vi "TRHmeasurement.vi"() -> ()   [LabVIEW 2018]
panel:
  in  "Instrument":enum16{"AG34401A", "Arduino", "Manually"}(ring)
  in  "rel. Humidity [%] in":dbl
  in  "Temperature [°C] in":dbl
  in  "Write into text file":bool
  in  "stop":bool
  in  "Measurement delay [s]":u32=5
  out "Rel. Humidity [%]":dbl
  out "Temperature [°C]":dbl
  out "Max temperature [°C]":dbl
  out "Min temperature [°C]":dbl
  out "Max RH [%]":dbl
  out "Min RH [%]":dbl
  out "Last 10 measurements":string[][](table)
  out "Temp. & RH":cluster{dbl[], dbl[]}[](graph)
  out "Average temperature [°C]":dbl
  out "Average RH [%]":dbl
  out "Iteration start time":timestamp
  out "time":string
  out "error out":errorcluster
  in  "T&RH":refnum<visa-resource-name>="COM4"
  in  "error in":errorcluster
  in  "Select folder to save data":path=path "C:/Users/itkstriplabview5/Documents"
  out "output file refnum":refnum<file>
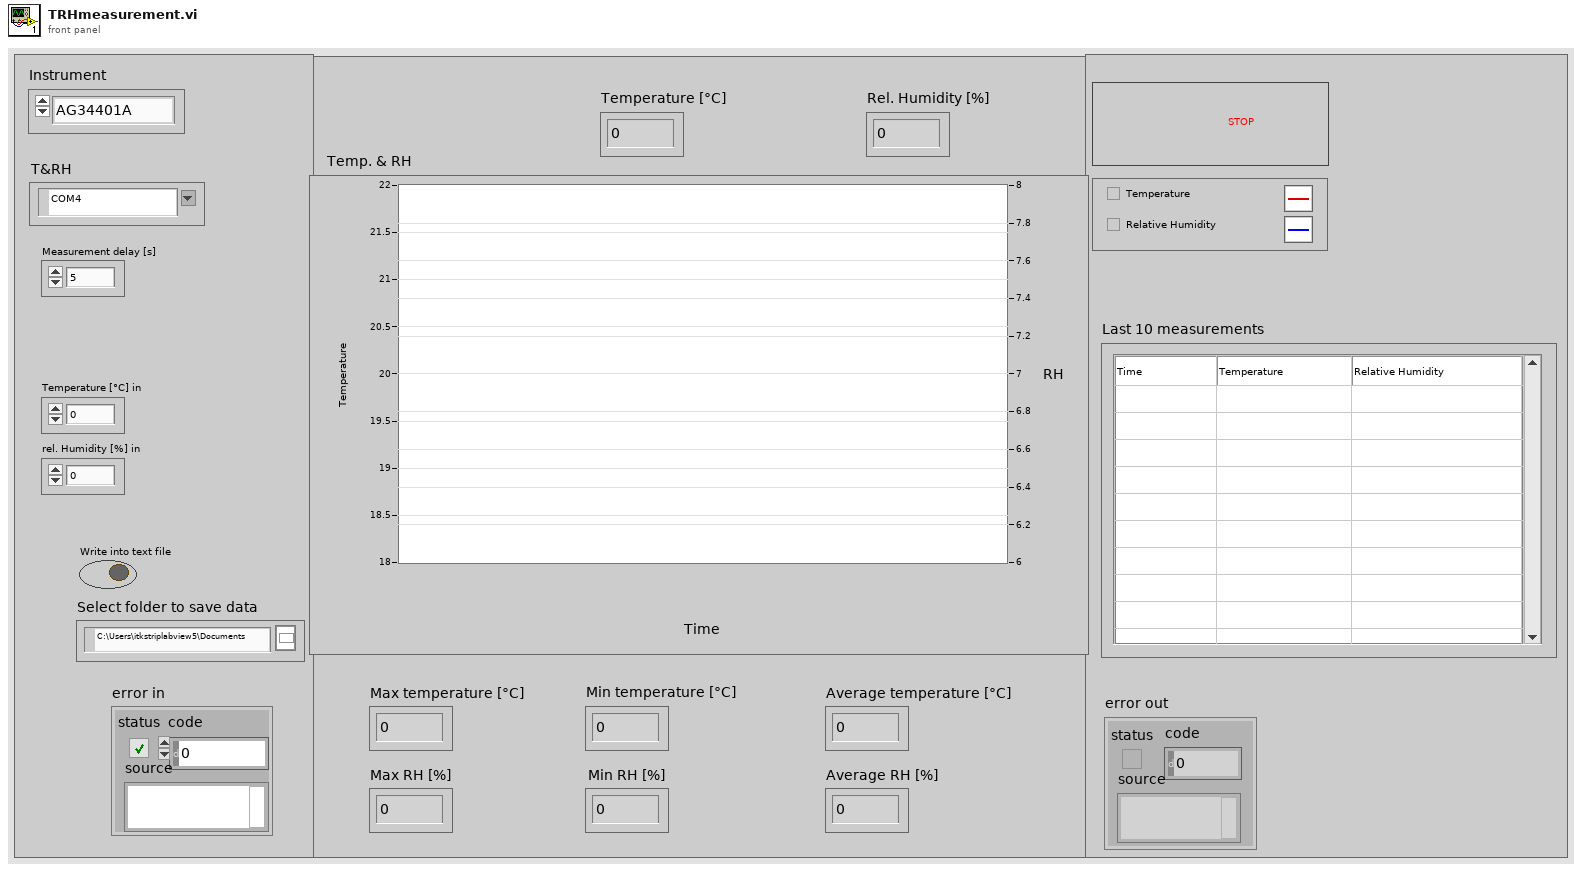
[diagram p1: front panel]
types:
  T1 = enum16{"open", "replace", "create", "open or create", "replace or create", "replace or create with confirmation"}
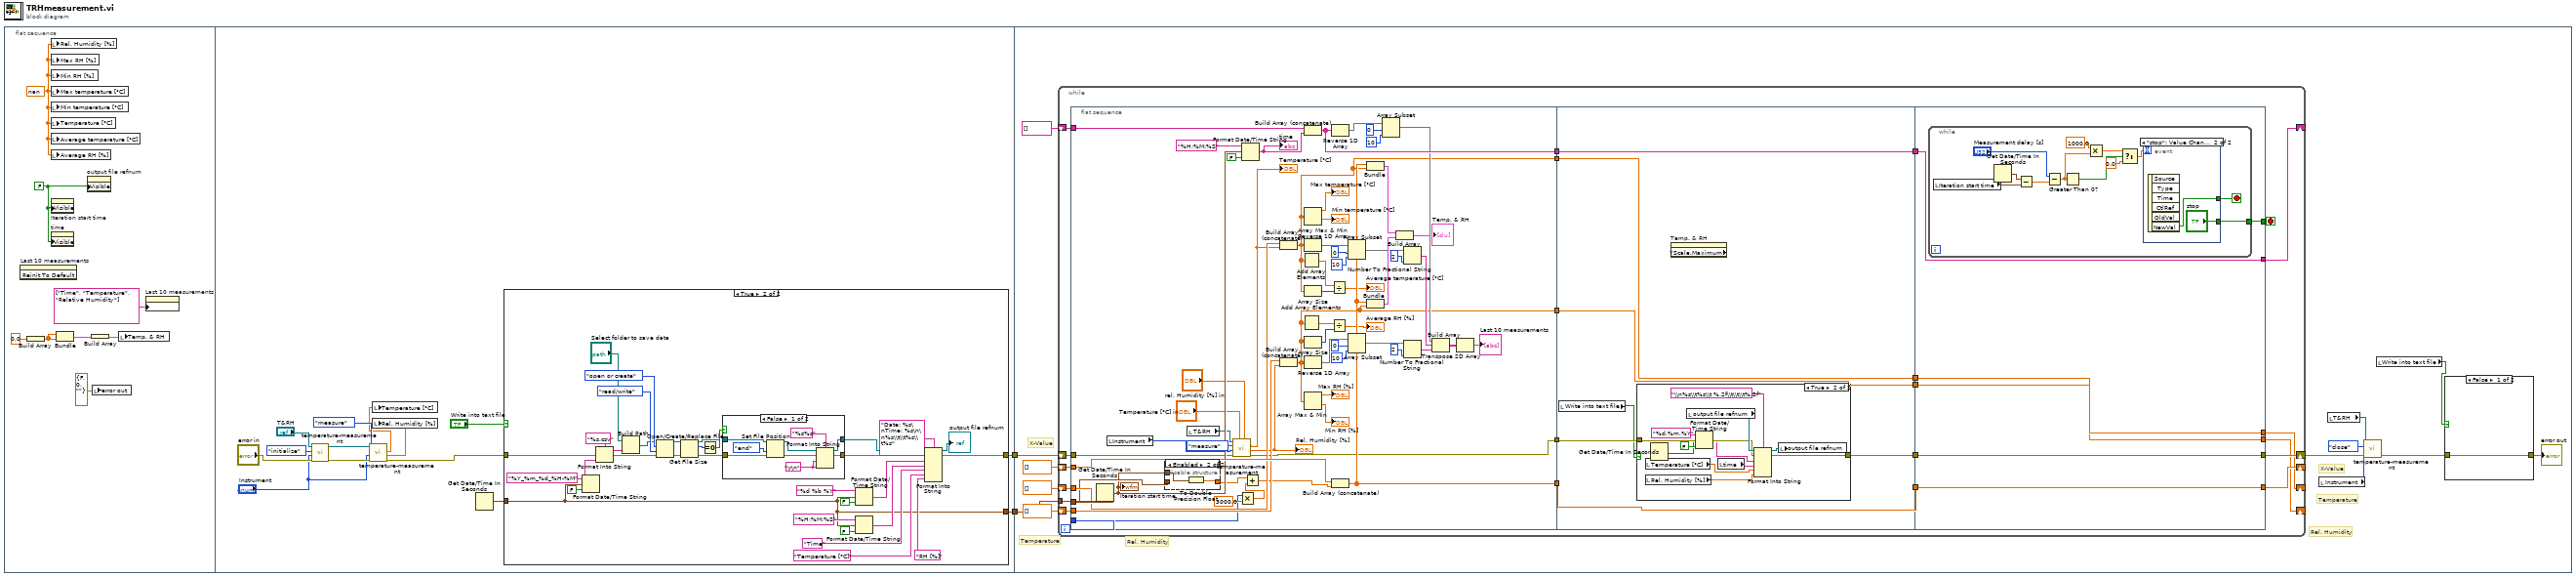
[diagram p0: block diagram]
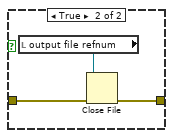
[diagram p4: hidden frame]
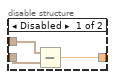
[diagram p5: hidden frame]
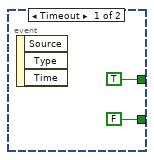
[diagram p7: hidden frame]
diagram:
  n1 = flat-sequence {
    tunnel: [w24] -> w2
    tunnel: [w23] -> w1
    tunnel: w2 -> [w78]
    tunnel: w1 -> [w76]
    frame #0 {
      w4 = FALSE ("Visible")
      w7 = nan
      n2 = invoke on="Last 10 measurements" class="Tbl (strict)" method="Reinit To Default"() -> ()  [unwired: 3 in, 3 out]
      n3 = Build Array(0.0) -> (w9:dbl[])
      n4 = local write "Rel. Humidity [%]"(w7) -> ()
      n5 = local write "Max RH [%]"(w7) -> ()
      n6 = local write "Min RH [%]"(w7) -> ()
      n7 = local write "Max temperature [°C]"(w7) -> ()
      n8 = local write "Min temperature [°C]"(w7) -> ()
      n9 = local write "Temperature [°C]"(w7) -> ()
      n10 = local write "Average temperature [°C]"(w7) -> ()
      n11 = local write "Average RH [%]"(w7) -> ()
      n12 = property on="Iteration start time" class="AbsTime (strict)"("Visible"=w4) -> ()  [unwired: 2 in, 2 out]
      n13 = property on="time" class="Str"("Visible"=w4) -> ()  [unwired: 2 in, 2 out]
      n14 = Bundle(w9, w9) -> (w8:cluster{dbl[], dbl[]})  [unwired: 1 in]
      n15 = property on="output file refnum" class="Ref (strict)"("Visible"=w4) -> ()  [unwired: 2 in, 2 out]
      n16 = Build Array(w8) -> (w10:cluster{dbl[], dbl[]}[])
      n17 = local write "error out"(errorcluster {"status"=FALSE, "code"=0, "source"=""} ("error out")) -> ()
      n18 = local write "Temp. & RH"(w10) -> ()
      n19 = property on="Last 10 measurements" class="Tbl (strict)"("Column Headers[]"=string[] ["Time", "Temperature", "Relative Humidity"]) -> ()  [unwired: 2 in, 2 out]
    }
    frame #1 {
      n20 = call "temperature-measurement.vi"("error in (no error)"="error in", "Instrument"="Instrument", "Action"=enum16{"initialize", "measure", "close"}."initialize", "Address (for temperature)"="T&RH") -> ("error out"=w16:errorcluster, "VISA resource name out"=w17:refnum<visa-resource-name>)  [unwired: 4 in, 2 out]
      n21 = call "temperature-measurement.vi"("error in (no error)"=w16, "Instrument"="Instrument", "Action"=enum16{"initialize", "measure", "close"}."measure", "Address (for temperature)"=w17) -> ("error out"=w11:errorcluster, "RH [%]"=w12:dbl, "T [°C]"=w13:dbl)  [unwired: 4 in, 1 out]
      n22 = local write "Temperature [°C]"(w13) -> ()
      n23 = local write "Rel. Humidity [%]"(w12) -> ()
      n24 = Get Date/Time In Seconds() -> (seconds since 1Jan1904=w21:timestamp)
      n25 = case shown="True" "Write into text file" {
        tunnel: [w26 w33] -> w24
        tunnel: w11 -> [w26 w28]
        tunnel: [w25 w27] -> w23
        tunnel: w21 -> [w25 w27]
        frame False {
        }
        frame True {
          n26 = Format Date/Time String(time format string (%c)="%Y_%m_%d_%H-%M", seconds (now)=w27, UTC format=FALSE) -> (date/time string=w41:string)
          n27 = Format Into String(format string="%s.csv", error in=w28, w41) -> (resulting string=w55:string, error out=w54:errorcluster)  [unwired: 1 in]
          n28 = Build Path(base path="Select folder to save data", name or relative path=w55) -> (appended path=w53:path)
          n29 = Open/Create/Replace File(file path (use dialog)=w53, error in=w54, operation (0:open)=T1."open or create", access (0:read/write)=enum16{"read/write", "read-only", "write-only"}."read/write") -> (refnum out=w51:refnum<file>, error out=w50:errorcluster)  [unwired: 2 in, 1 out]
          n30 = Get File Size(file=w51, error in=w50) -> (refnum out=w47:refnum<file>, size (in bytes)=w49:i64, 0:w46:errorcluster)
          n31 = Equal To 0?(x=w49) -> (x = 0?=w48:bool)
          n32 = case shown="False" w48 {
            tunnel: w47 -> [w67 w69]
            tunnel: w46 -> [w66 w68]
            tunnel: [w61 w69] -> w44
            tunnel: [w60 w68] -> w45
            frame False {
              w59 = "\r\n"
              n33 = Set File Position(refnum=w67, from (0:start)=enum16{"start", "end", "current"}."end", error in=w66) -> (refnum out=w63:refnum<file>, error out=w62:errorcluster)  [unwired: 1 in]
              n34 = Format Into String(format string="%s%s", initial string=w63, error in=w62, w59, w59) -> (resulting string=w61:refnum<file>, error out=w60:errorcluster)
            }
            frame True {
            }
          }
          n35 = Format Date/Time String(time format string (%c)="%d %b %Y", seconds (now)=w27, UTC format=FALSE) -> (date/time string=w38:string)
          n36 = Format Date/Time String(time format string (%c)="%H:%M:%S", seconds (now)=w27, UTC format=FALSE) -> (date/time string=w35:string)
          n37 = Format Into String(format string="Date: %s\nTime: %s\n\n%s\\t\\t%s\\t%s", initial string=w44, error in=w45, w38, w35, "Time" ("input 3"), "Temperature [°C]" ("input 4"), "RH [%]" ("input 5")) -> (resulting string=→"output file refnum":refnum<file>, error out=w33:errorcluster)
        }
      }
    }
    frame #2 {
      # "Rel. Humidity"
      # "Temperature"
      # "X-Value"
      # "Rel. Humidity"
      # "Temperature"
      # "X-Value"
      n38 = while {
        shift-right: [w109] -> w74
        shift-left: w78 -> [w105]
        shift-right: [w104] -> _
        shift-left: dbl[] [] -> [w108]
        shift-right: [w101] -> _
        shift-left: dbl[] [] -> [w107]
        shift-right: [w100] -> _
        shift-left: dbl[] [] -> [w106]
        shift-right: [w102] -> _
        shift-left: string[] [] -> [w103]
        tunnel: w76 -> [w88]
        i -> [w87]
        stop <- w99 stop-if-true
        n39 = flat-sequence {
          tunnel: w108 -> [w167]
          tunnel: w107 -> [w166]
          tunnel: w106 -> [w165]
          tunnel: w105 -> [w118]
          tunnel: w103 -> [w147]
          tunnel: [w158] -> w97
          tunnel: [w143] -> w95
          tunnel: [w134] -> w93
          tunnel: [w130] -> w91
          tunnel: [w117] -> w89
          tunnel: w88 -> [w125]
          tunnel: w87 -> [w122]
          tunnel: [w175] -> w98
          tunnel: w97 -> [w179]
          tunnel: [w179] -> w96
          tunnel: w95 -> [w178]
          tunnel: [w178] -> w94
          tunnel: w93 -> [w177]
          tunnel: [w177] -> w92
          tunnel: w91 -> [w176]
          tunnel: [w176] -> w90
          tunnel: w89 -> [w174]
          tunnel: [w194] -> w100
          tunnel: [w195] -> w101
          tunnel: [w196] -> w102
          tunnel: [w197] -> w104
          tunnel: [w198] -> w109
          tunnel: w98 -> [w198]
          tunnel: w96 -> [w197]
          tunnel: w94 -> [w196]
          tunnel: w92 -> [w195]
          tunnel: w90 -> [w194]
          tunnel: [w193] -> w99
          frame #0 {
            n40 = Get Date/Time In Seconds() -> (seconds since 1Jan1904=w124:timestamp)
            "Iteration start time" <- w124
            n41 = local read "Instrument"() -> (w111:enum16{"AG34401A", "Arduino", "Manually"})
            n42 = disable-structure shown="Enabled" {
              disable-tunnel: w125 -> [w170 _]
              disable-tunnel: [w169 w172] -> w121
              disable-tunnel: w124 -> [w168 w171]
              frame Disabled {
                n43 = Subtract(x=w168, y=w170) -> (x-y=w169:dbl)
              }
              frame Enabled {
                n44 = To Double Precision Float(number=w171) -> (double precision float=w172:dbl)
              }
            }
            n45 = local read "T&RH"() -> (w110:refnum<visa-resource-name>)
            n46 = call "temperature-measurement.vi"("Enter RH [%]"="rel. Humidity [%] in", "Enter temp. [°C]"="Temperature [°C] in", "error in (no error)"=w118, "Instrument"=w111, "Action"=enum16{"initialize", "measure", "close"}."measure", "Address (for temperature)"=w110) -> ("error out"=w117:errorcluster, "RH [%]"=w114:dbl, "T [°C]"=w113:dbl)  [unwired: 2 in, 1 out]
            "Rel. Humidity [%]" <- w114
            "Temperature [°C]" <- w113
            n47 = Multiply(x=w122, y=3000.0) -> (x*y=w120:dbl)
            n48 = Format Date/Time String(time format string (%c)="%H:%M:%S", seconds (now)=w124, UTC format=FALSE) -> (date/time string=w127:string)
            "time" <- w127
            n49 = Add(x=w121, y=w120) -> (x+y=w119:dbl)
            n50 = Build Array (concatenate)(w166, w113) -> (w134:dbl[])
            n51 = Build Array (concatenate)(w165, w114) -> (w130:dbl[])
            n52 = Add Array Elements(numeric array=w134) -> (sum=w135:dbl)
            n53 = Add Array Elements(numeric array=w130) -> (sum=w131:dbl)
            n54 = Build Array (concatenate)(w147, w127) -> (w143:string[])
            n55 = Array Max & Min(array=w134) -> (max value=→"Max temperature [°C]":dbl, min value=→"Min temperature [°C]":dbl)  [unwired: 2 out]
            n56 = Reverse 1D Array(array=w134) -> (reversed array=w155:dbl[])
            n57 = Array Size(array=w134) -> (size(s)=w136:i32)
            n58 = Array Size(array=w130) -> (size(s)=w132:i32)
            n59 = Reverse 1D Array(array=w130) -> (reversed array=w152:dbl[])
            n60 = Array Max & Min(array=w130) -> (max value=→"Max RH [%]":dbl, min value=→"Min RH [%]":dbl)  [unwired: 2 out]
            n61 = Divide(x=w135, y=w136) -> (x/y=→"Average temperature [°C]":dbl)
            n62 = Divide(x=w131, y=w132) -> (x/y=→"Average RH [%]":dbl)
            n63 = Reverse 1D Array(array=w143) -> (reversed array=w144:string[])
            n64 = Build Array (concatenate)(w167, w119) -> (w158:dbl[])
            n65 = Array Subset(array=w155, index=0, length=10) -> (w149:dbl[])
            n66 = Array Subset(array=w152, index=0, length=10) -> (w151:dbl[])
            n67 = Bundle(w158, w134) -> (w164:cluster{dbl[], dbl[]})  [unwired: 1 in]
            n68 = Bundle(w158, w130) -> (w163:cluster{dbl[], dbl[]})  [unwired: 1 in]
            n69 = Array Subset(array=w144, index=0, length=10) -> (w142:string[])
            n70 = Build Array(w164, w163) -> (→"Temp. & RH":cluster{dbl[], dbl[]}[])
            n71 = Number To Fractional String(number=w149, precision (6)=i16 2) -> (F-format string=w141:string[])  [unwired: 2 in]
            n72 = Number To Fractional String(number=w151, precision (6)=i16 2) -> (F-format string=w140:string[])  [unwired: 2 in]
            n73 = Build Array(w142, w141, w140) -> (w139:string[][])
            n74 = Transpose 2D Array(2D array=w139) -> (transposed array=→"Last 10 measurements":string[][])
          }
          frame #1 {
            n75 = local read "Write into text file"() -> (w173:bool)
            n76 = case shown="True" w173 {
              tunnel: [w180 w189] -> w175
              tunnel: w174 -> [w180 w186]
              frame False {
              }
              frame True {
                n77 = local read "Temperature [°C]"() -> (w191:dbl)
                n78 = local read "Rel. Humidity [%]"() -> (w190:dbl)
                n79 = Get Date/Time In Seconds() -> (seconds since 1Jan1904=w183:timestamp)
                n80 = local read "output file refnum"() -> (w187:refnum<file>)
                n81 = Format Date/Time String(time format string (%c)="%d.%m.%Y", seconds (now)=w183, UTC format=FALSE) -> (date/time string=w181:string)
                n82 = local read "time"() -> (w182:string)
                n83 = Format Into String(format string="\\n%s\\t%s\\t %.2f\\t\\t\\t%.2f", initial string=w187, error in=w186, w181, w182, w191, w190) -> (resulting string=w188:refnum<file>, error out=w189:errorcluster)
                n84 = local write "output file refnum"(w188) -> ()
              }
            }
            n85 = property on="Temp. & RH" class="XYGraph (strict)" props=["YScale", "Maximum"]() -> ()  [unwired: 2 in, 3 out]
          }
          frame #2 {
            n86 = while {
              tunnel: [w199] -> w193
              stop <- w200 stop-if-true
              n87 = local read "Iteration start time"() -> (w209:timestamp)
              n88 = Get Date/Time In Seconds() -> (seconds since 1Jan1904=w210:timestamp)
              n89 = Subtract(x=w210, y=w209) -> (x-y=w207:dbl)
              n90 = Subtract(x="Measurement delay [s]", y=w207) -> (x-y=w204:dbl)
              n91 = Greater Than 0?(x=w204) -> (x > 0?=w206:bool)
              n92 = Multiply(x=1000.0, y=w204) -> (x*y=w202:dbl)
              n93 = Select(t=w202, s=w206, f=0.0) -> (s? t:f=w201:dbl)
              n94 = event shown="[1] \"stop\": Value Change" {
                selector: _ -> [_ _]
                dyn-events: _ -> [_ _]
                timeout: w201 -> [_ _]
                tunnel: [TRUE w214] -> w200
                tunnel: [FALSE "stop"] -> w199
                event Timeout {
                  n95 = event-data() -> ()  [unwired: 1 in, 3 out]
                }
                event "stop": Value Change {
                  n96 = event-data() -> ("NewVal"=w214:bool)  [unwired: 1 in, 5 out]
                }
              }
            }
          }
        }
      }
      n97 = local read "Instrument"() -> (w71:enum16{"AG34401A", "Arduino", "Manually"})
      n98 = local read "T&RH"() -> (w70:refnum<visa-resource-name>)
      n99 = call "temperature-measurement.vi"("error in (no error)"=w74, "Instrument"=w71, "Action"=enum16{"initialize", "measure", "close"}."close", "Address (for temperature)"=w70) -> ("error out"=w73:errorcluster)  [unwired: 4 in, 3 out]
      n100 = local read "Write into text file"() -> (w75:bool)
      n101 = case shown="False" w75 {
        tunnel: w73 -> [w83 w86]
        tunnel: [w83 w85] -> w77
        frame False {
        }
        frame True {
          n102 = local read "output file refnum"() -> (w84:refnum<file>)
          n103 = Close File(refnum=w84, error in=w86) -> (error out=w85:errorcluster)  [unwired: 1 out]
        }
      }
      "error out" <- w77
    }
  }
